vi "Can_Be_Package_Top_Level.vi"(8 "error in (no error)":errorcluster, 9 "AB_Source in":refnum<class "AB_Source.lvclass">, 11 "Build in":refnum<class "AB_Build.lvclass">) -> (0 "error out":errorcluster, 2 "topLevel":bool, 3 "Build out":refnum<class "AB_Build.lvclass">)   [LabVIEW 2020, in "AB_Build.lvclass"]
uses:
  <vilib>/AppBuilder/AB_Classes/Build/AB_Build.lvclass
  <vilib>/AppBuilder/AB_Classes/Source/AB_Source.lvclass
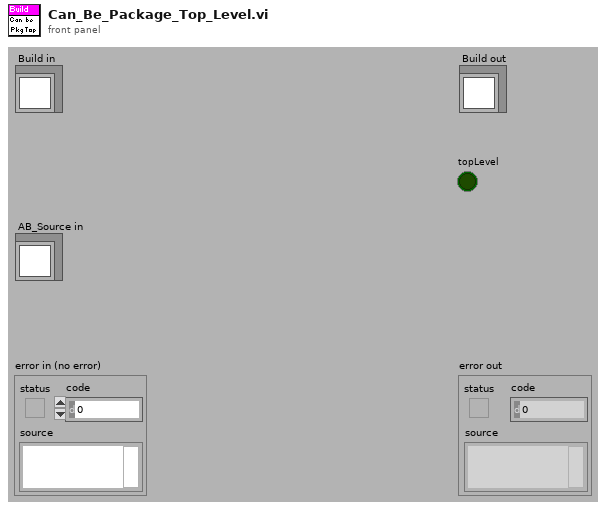
[diagram p1: front panel]
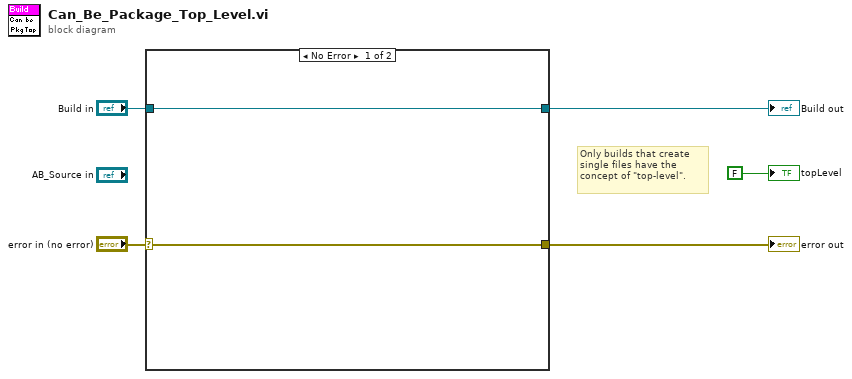
[diagram p0: block diagram]
diagram:
  # "Only builds that create single files have the concept of \"top-level\"."
  n1 = case shown="No Error" "error in (no error)" {
    selector: "error in (no error)" -> [w7 w9]
    tunnel: [w7 w9] -> w4
    tunnel: [w6 w8] -> w2
    tunnel: "Build in" -> [w6 w8]
    frame No Error {
    }
    frame Error {
    }
  }
  "error out" <- w4
  "Build out" <- w2
  "topLevel" <- FALSE
